vi "Calibration (SubVI).vi"(0 "PT-FU-120 (INPUT)":dbl, 1 "PT-OX-210 (INPUT)":dbl, 2 "PT-OX-220 (INPUT)":dbl, 3 "PT-FU-310 (INPUT)":dbl, 4 "PT-FU-320 (INPUT)":dbl, 5 "PT-CC-410 (INPUT)":dbl, 6 "PT-OX-130 (INPUT)":dbl, 7 "LC-OX-210 (INPUT)":dbl, 8 "PT-PR-110 (INPUT)":dbl, 9 "LC-FU-310 (INPUT)":dbl) -> (10 "PT-PR-110 (OUTPUT)":dbl, 11 "PT-CC-410 (OUTPUT)":dbl, 12 "PT-OX-130 (OUTPUT)":dbl, 13 "LC-FU-310 (OUTPUT)":dbl, 14 "PT-FU-120 (OUTPUT)":dbl, 15 "PT-OX-210 (OUTPUT)":dbl, 16 "PT-OX-220 (OUTPUT)":dbl, 17 "PT-FU-310 (OUTPUT":dbl, 18 "PT-FU-320 (OUTPUT)":dbl, 19 "LC-OX-210 (OUTPUT)":dbl)   [LabVIEW 2020]
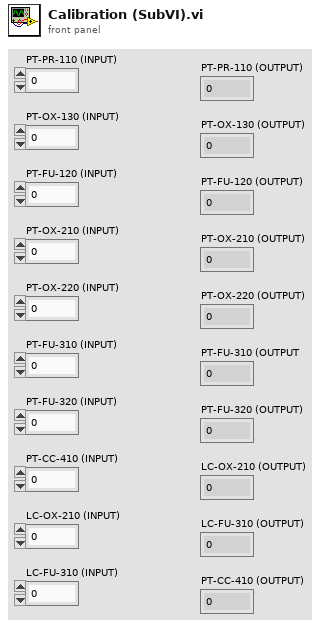
[diagram p1: front panel]
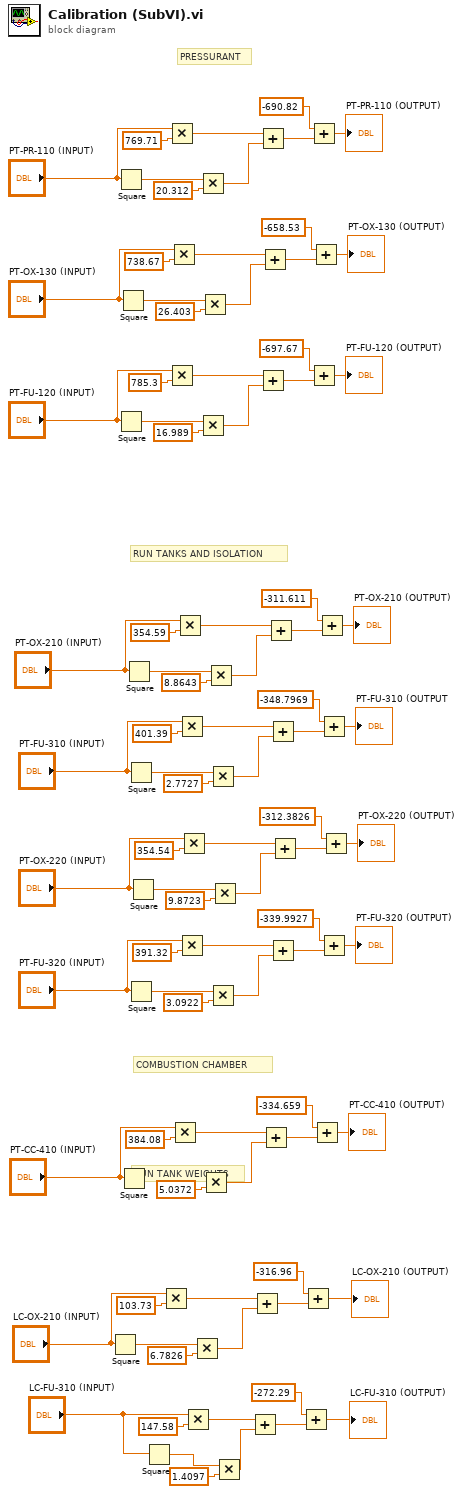
[diagram p0: block diagram]
diagram:
  # "RUN TANK WEIGHTS"
  # "COMBUSTION CHAMBER"
  # "RUN TANKS AND ISOLATION"
  # "PRESSURANT"
  n1 = Square(x="LC-OX-210 (INPUT)") -> (x^2=w15:dbl)
  n2 = Square(x="PT-PR-110 (INPUT)") -> (x^2=w87:dbl)
  n3 = Square(x="PT-FU-120 (INPUT)") -> (x^2=w69:dbl)
  n4 = Square(x="PT-OX-130 (INPUT)") -> (x^2=w78:dbl)
  n5 = Square(x="PT-CC-410 (INPUT)") -> (x^2=w29:dbl)
  n6 = Square(x="PT-OX-210 (INPUT)") -> (x^2=w62:dbl)
  n7 = Square(x="PT-FU-310 (INPUT)") -> (x^2=w48:dbl)
  n8 = Square(x="PT-FU-320 (INPUT)") -> (x^2=w41:dbl)
  n9 = Square(x="PT-OX-220 (INPUT)") -> (x^2=w55:dbl)
  n10 = Square(x="LC-FU-310 (INPUT)") -> (x^2=w8:dbl)
  n11 = Multiply(x="LC-OX-210 (INPUT)", y=103.73) -> (x*y=w13:dbl)
  n12 = Multiply(x="PT-PR-110 (INPUT)", y=769.71) -> (x*y=w85:dbl)
  n13 = Multiply(x="PT-FU-120 (INPUT)", y=785.3) -> (x*y=w67:dbl)
  n14 = Multiply(x="PT-OX-130 (INPUT)", y=738.67) -> (x*y=w76:dbl)
  n15 = Multiply(x="PT-CC-410 (INPUT)", y=384.08) -> (x*y=w27:dbl)
  n16 = Multiply(x="PT-OX-210 (INPUT)", y=354.59) -> (x*y=w60:dbl)
  n17 = Multiply(x="PT-FU-310 (INPUT)", y=401.39) -> (x*y=w46:dbl)
  n18 = Multiply(x="PT-FU-320 (INPUT)", y=391.32) -> (x*y=w39:dbl)
  n19 = Multiply(x="PT-OX-220 (INPUT)", y=354.54) -> (x*y=w53:dbl)
  n20 = Multiply(x="LC-FU-310 (INPUT)", y=147.58) -> (x*y=w6:dbl)
  n21 = Multiply(x=w15, y=6.7826) -> (x*y=w14:dbl)
  n22 = Multiply(x=w87, y=20.312) -> (x*y=w86:dbl)
  n23 = Multiply(x=w69, y=16.989) -> (x*y=w68:dbl)
  n24 = Multiply(x=w78, y=26.403) -> (x*y=w77:dbl)
  n25 = Multiply(x=w29, y=5.0372) -> (x*y=w28:dbl)
  n26 = Multiply(x=w62, y=8.8643) -> (x*y=w61:dbl)
  n27 = Multiply(x=w48, y=2.7727) -> (x*y=w47:dbl)
  n28 = Multiply(x=w41, y=3.0922) -> (x*y=w40:dbl)
  n29 = Multiply(x=w55, y=9.8723) -> (x*y=w54:dbl)
  n30 = Multiply(x=w8, y=1.4097) -> (x*y=w7:dbl)
  n31 = Add(x=w6, y=w7) -> (x+y=w5:dbl)
  n32 = Add(x=w13, y=w14) -> (x+y=w12:dbl)
  n33 = Add(x=w85, y=w86) -> (x+y=w84:dbl)
  n34 = Add(x=w67, y=w68) -> (x+y=w66:dbl)
  n35 = Add(x=w76, y=w77) -> (x+y=w75:dbl)
  n36 = Add(x=w27, y=w28) -> (x+y=w26:dbl)
  n37 = Add(x=w60, y=w61) -> (x+y=w59:dbl)
  n38 = Add(x=w46, y=w47) -> (x+y=w45:dbl)
  n39 = Add(x=w39, y=w40) -> (x+y=w38:dbl)
  n40 = Add(x=w53, y=w54) -> (x+y=w52:dbl)
  n41 = Add(x=-272.29, y=w5) -> (x+y=→"LC-FU-310 (OUTPUT)":dbl)
  n42 = Add(x=-316.96, y=w12) -> (x+y=→"LC-OX-210 (OUTPUT)":dbl)
  n43 = Add(x=-690.82, y=w84) -> (x+y=→"PT-PR-110 (OUTPUT)":dbl)
  n44 = Add(x=-697.67, y=w66) -> (x+y=→"PT-FU-120 (OUTPUT)":dbl)
  n45 = Add(x=-658.53, y=w75) -> (x+y=→"PT-OX-130 (OUTPUT)":dbl)
  n46 = Add(x=-334.659, y=w26) -> (x+y=→"PT-CC-410 (OUTPUT)":dbl)
  n47 = Add(x=-311.611, y=w59) -> (x+y=→"PT-OX-210 (OUTPUT)":dbl)
  n48 = Add(x=-348.7969, y=w45) -> (x+y=→"PT-FU-310 (OUTPUT":dbl)
  n49 = Add(x=-339.9927, y=w38) -> (x+y=→"PT-FU-320 (OUTPUT)":dbl)
  n50 = Add(x=-312.3826, y=w52) -> (x+y=→"PT-OX-220 (OUTPUT)":dbl)
